vi "lockinOptimiser_old.vi"() -> ()   [LabVIEW 2014]
uses:
  <vilib>/Utility/file.llb/Read From Spreadsheet File (DBL).vi
  <userlib>/Nanonis Prog Interface V5/Nanonis Prog Interface.lvlib
  <vilib>/Analysis/NI_AALBase.lvlib
panel:
  in  "stop":bool
  in  "Start":bool
  in  "Clear Chart":bool
  in  "End Index":dbl=351.0
  in  "Start Index":dbl=250.0
  out "SNR":cluster{"all rows":dbl[], dbl[]}[](graph)
  out "Demod":cluster{"all rows":dbl[], dbl[]}[](graph)
  out "Std Dev Demod":cluster{"all rows":dbl[], dbl[]}[](graph)
  in  "Settling Time (ms)":i32=1000
  in  "Integration Time (ms)":i32=600
  out "all rows":dbl[][](array[numeric]) format="%0.3f"
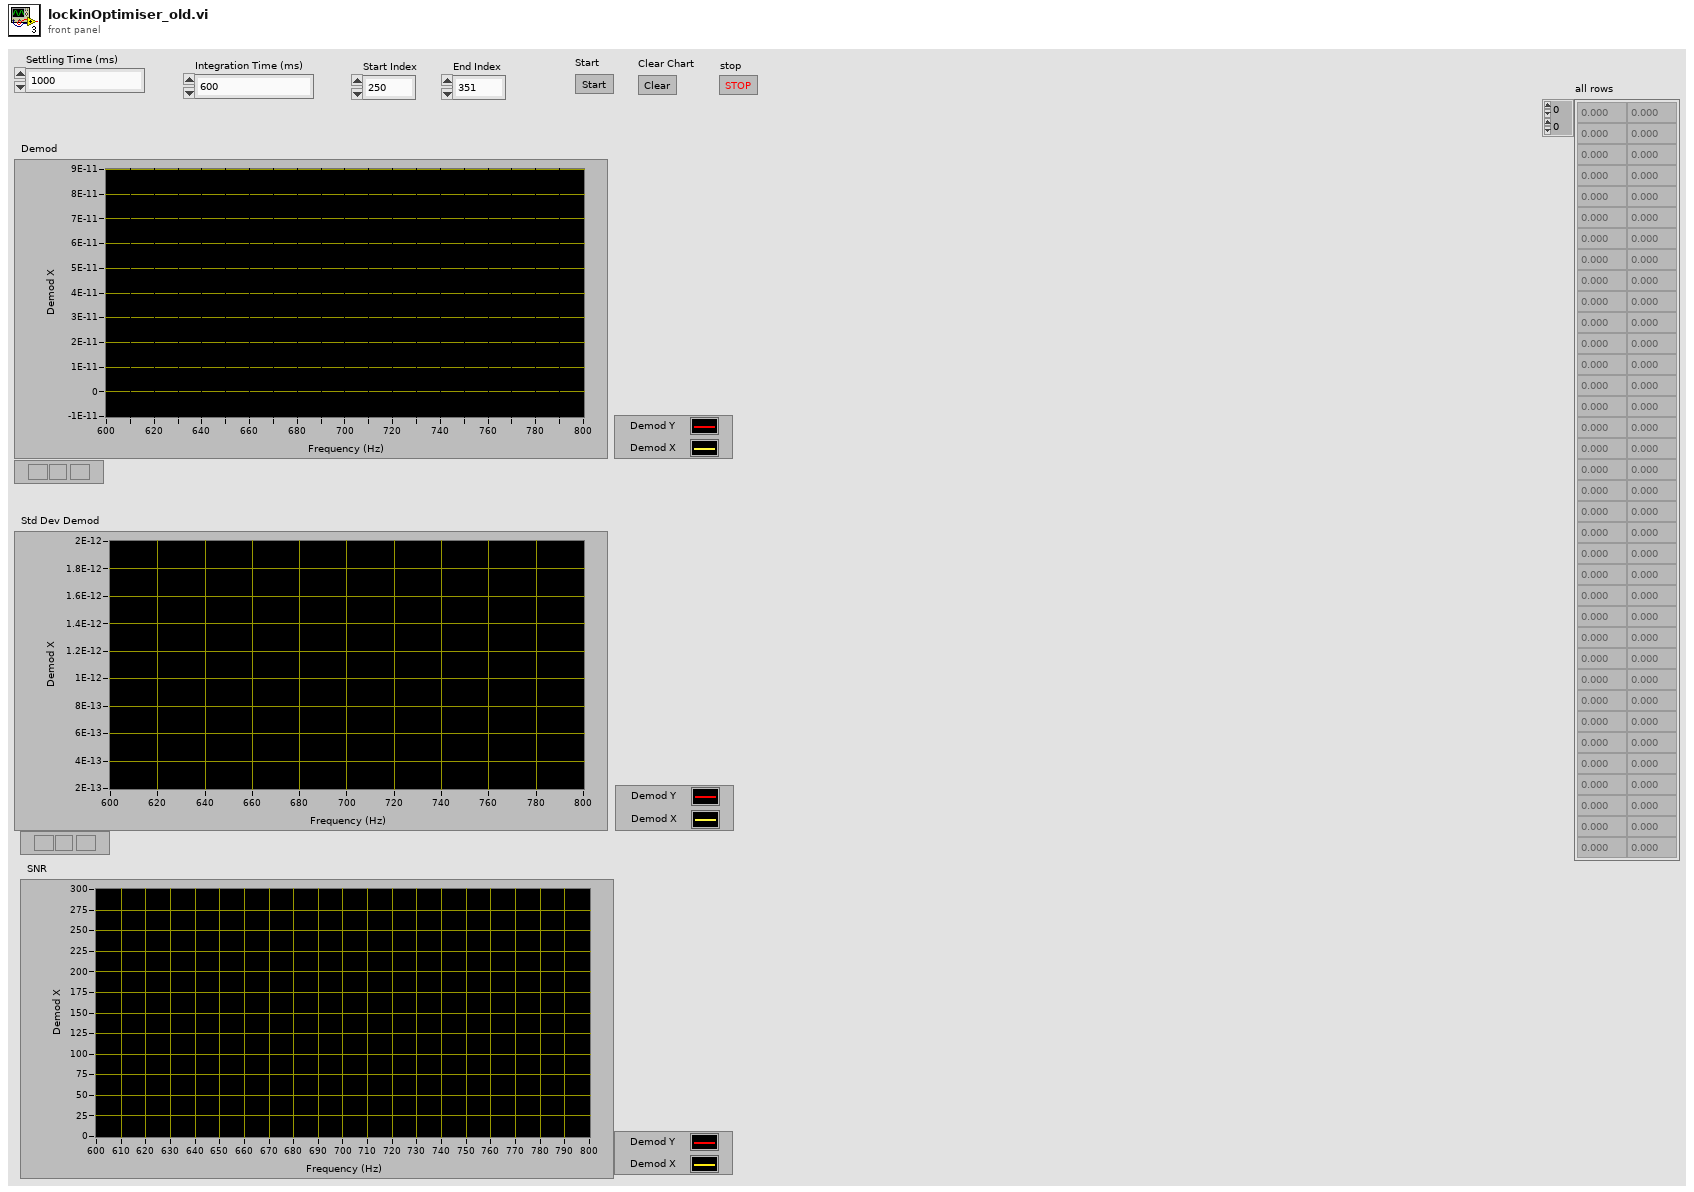
[diagram p1: front panel]
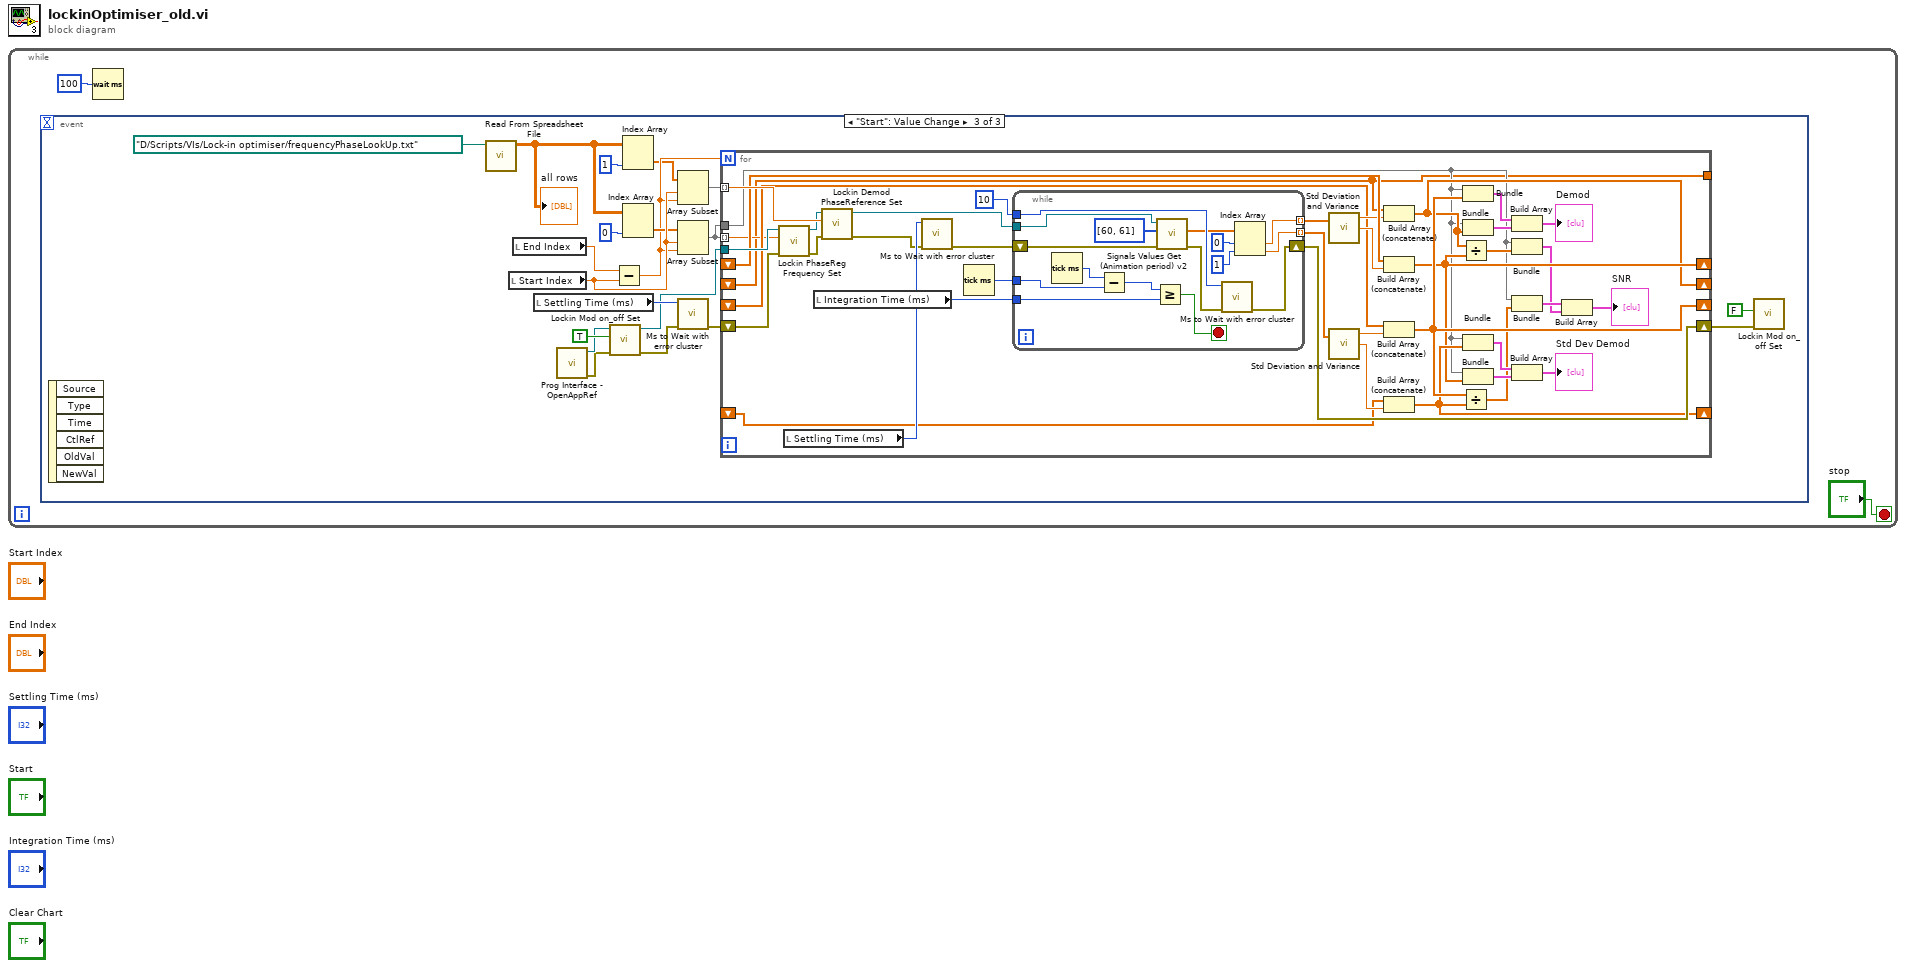
[diagram p0: block diagram]
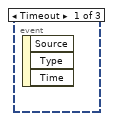
[diagram p2: hidden frame]
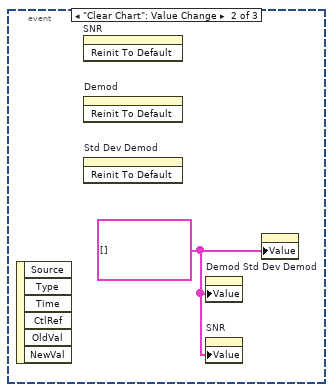
[diagram p3: hidden frame]
diagram:
  n1 = while {
    stop <- "stop" stop-if-true
    n2 = event shown="[2] \"Start\": Value Change" {
      selector: _ -> [_ _ _]
      dyn-events: _ -> [_ _ _]
      timeout: _ -> [_ _ _]
      event Timeout {
        n3 = event-data() -> ()  [unwired: 1 in, 3 out]
      }
      event "Clear Chart": Value Change {
        w3 = cluster{"all rows":dbl[], dbl[]}[] [] ("Demod")
        n4 = event-data() -> ()  [unwired: 1 in, 6 out]
        n5 = invoke on="SNR" class="XYGraph (strict)" method="Reinit To Default"() -> ()  [unwired: 3 in, 3 out]
        n6 = invoke on="Demod" class="XYGraph (strict)" method="Reinit To Default"() -> ()  [unwired: 3 in, 3 out]
        n7 = invoke on="Std Dev Demod" class="XYGraph (strict)" method="Reinit To Default"() -> ()  [unwired: 3 in, 3 out]
        n8 = property on="Demod" class="XYGraph (strict)"("Value"=w3) -> ()  [unwired: 2 in, 2 out]
        n9 = property on="SNR" class="XYGraph (strict)"("Value"=w3) -> ()  [unwired: 2 in, 2 out]
        n10 = property on="Std Dev Demod" class="XYGraph (strict)"("Value"=w3) -> ()  [unwired: 2 in, 2 out]
      }
      event "Start": Value Change {
        n11 = event-data() -> ()  [unwired: 1 in, 6 out]
        n12 = call-poly <vilib>:"Read From Spreadsheet File.vi"("file path (dialog if empty)"=path "D:/Scripts/VIs/Lock-in optimiser/frequencyPhaseLookUp.txt") -> ("all rows"=w7:dbl[][])  [unwired: 6 in, 4 out]
        "all rows" <- w7
        n13 = local read "Start Index"() -> (w22:dbl)
        n14 = local read "End Index"() -> (w23:dbl)
        n15 = local read "Settling Time (ms)"() -> (w21:i32)
        n16 = call <userlib>:"Prog Interface - OpenAppRef.vi"() -> ("Error out"=w8:errorcluster, "Application reference"=w9:refnum<vi>)  [unwired: 6 in]
        n17 = call <userlib>:"Lockin Mod on_off Set.vi"("Error in (no error)"=w8, "Lockin ON/OFF"=TRUE, "Application ref in"=w9) -> ("Error out"=w11:errorcluster, "Application ref out"=w10:refnum<vi>)  [unwired: 7 in]
        n18 = Subtract(x=w23, y=w22) -> (x-y=w17:dbl)
        n19 = Index Array(array=w7, index (col)=1 ("index")) -> (element=w16:dbl[])  [unwired: 1 in]
        n20 = Index Array(array=w7, index (col)=0 ("index")) -> (element=w18:dbl[])  [unwired: 1 in]
        n21 = Array Subset(array=w16, index=w22, length=w17) -> (w20:dbl[])
        n22 = Array Subset(array=w18, index=w22, length=w17) -> (w19:dbl[])
        n23 = call <userlib>:"Ms to Wait with error cluster.vi"("error in (no error)"=w11, "milliseconds to wait"=w21) -> ("error out"=w12:errorcluster)  [unwired: 4 in, 1 out]
        n24 = for {
          N: w17 -> [_]
          tunnel: w19 -> [w41] mode=indexing
          tunnel: w20 -> [w63] mode=indexing
          tunnel: w10 -> [w62]
          shift-right: [w51] -> w14
          shift-left: w12 -> [w60]
          shift-right: [w32] -> _
          shift-left: _ -> [w48]
          shift-right: [w31] -> _
          shift-left: _ -> [w24]
          shift-right: [w34] -> _
          shift-left: _ -> [w44]
          shift-right: [w33] -> _
          shift-left: _ -> [w42]
          tunnel: w19 -> [w28]
          tunnel: [w24] -> _
          n25 = call <userlib>:"Lockin PhaseReg Frequency Set.vi"("Error in (no error)"=w60, "Frequency (Hz)"=w41, "Application ref in"=w62) -> ("Error out"=w59:errorcluster, "Application ref out"=w61:refnum<vi>)  [unwired: 7 in]
          n26 = local read "Settling Time (ms)"() -> (w54:i32)
          n27 = local read "Integration Time (ms)"() -> (w55:i32)
          n28 = call <userlib>:"Lockin Demod PhaseReference Set.vi"("Error in (no error)"=w59, "Phase Reference"=w63, "Application ref in"=w61) -> ("Error out"=w53:errorcluster, "Application ref out"=w52:refnum<vi>)  [unwired: 7 in]
          n29 = call <userlib>:"Ms to Wait with error cluster.vi"("error in (no error)"=w53, "milliseconds to wait"=w54) -> ("error out"=w58:errorcluster)  [unwired: 4 in, 1 out]
          n30 = Tick Count (ms)() -> (millisecond timer value=w57:u32)
          n31 = while {
            tunnel: w57 -> [w79]
            tunnel: 10 ("Integration Time (ms)") -> [w75]
            tunnel: w55 -> [w74]
            tunnel: w52 -> [w72]
            tunnel: [w65] -> w50 mode=indexing
            tunnel: [w64] -> w49 mode=indexing
            shift-right: [w73] -> w51
            shift-left: w58 -> [w71]
            stop <- w76 stop-if-true
            n32 = Tick Count (ms)() -> (millisecond timer value=w78:u32)
            n33 = Subtract(x=w78, y=w79) -> (x-y=w77:u32)
            n34 = Greater Or Equal?(x=w77, y=w74) -> (x >= y?=w76:bool)
            n35 = call <userlib>:"Signals Values Get (Animation period) v2.vi"("error in (no error)"=w71, "Signals indexes (0-79)"=i8[] [60, 61], "Application ref in"=w72) -> ("error out"=w70:errorcluster, "Signals Values"=w68:sgl[])  [unwired: 5 in, 1 out]
            n36 = call <userlib>:"Ms to Wait with error cluster.vi"("error in (no error)"=w70, "milliseconds to wait"=w75) -> ("error out"=w73:errorcluster)  [unwired: 4 in, 1 out]
            n37 = Index Array(array=w68, index #1=0 ("index"), index #2=1 ("index")) -> (element #1=w65:sgl, element #2=w64:sgl)
          }
          n38 = call <vilib>:"Std Deviation and Variance.vi"("X"=w50) -> ("mean"=w46:dbl, "standard deviation"=w47:dbl)  [unwired: 1 in, 1 out]
          n39 = call <vilib>:"Std Deviation and Variance.vi"("X"=w49) -> ("mean"=w45:dbl, "standard deviation"=w43:dbl)  [unwired: 1 in, 1 out]
          n40 = Build Array (concatenate)(w24, w46) -> (w31:dbl[])
          n41 = Build Array (concatenate)(w48, w47) -> (w32:dbl[])
          n42 = Build Array (concatenate)(w44, w45) -> (w34:dbl[])
          n43 = Build Array (concatenate)(w42, w43) -> (w33:dbl[])
          n44 = Divide(x=w31, y=w32) -> (x/y=w29:dbl[])
          n45 = Divide(x=w34, y=w33) -> (x/y=w30:dbl[])
          n46 = Bundle(w28, w34) -> (w39:cluster{dbl[], dbl[]})  [unwired: 1 in]
          n47 = Bundle(w28, w31) -> (w38:cluster{dbl[], dbl[]})  [unwired: 1 in]
          n48 = Bundle(w28, w33) -> (w36:cluster{dbl[], dbl[]})  [unwired: 1 in]
          n49 = Bundle(w28, w32) -> (w37:cluster{dbl[], dbl[]})  [unwired: 1 in]
          n50 = Build Array(w39, w38) -> (→"Demod":cluster{dbl[], dbl[]}[])
          n51 = Bundle(w28, w29) -> (w26:cluster{dbl[], dbl[]})  [unwired: 1 in]
          n52 = Bundle(w28, w30) -> (w27:cluster{dbl[], dbl[]})  [unwired: 1 in]
          n53 = Build Array(w36, w37) -> (→"Std Dev Demod":cluster{dbl[], dbl[]}[])
          n54 = Build Array(w27, w26) -> (→"SNR":cluster{dbl[], dbl[]}[])
        }
        n55 = call <userlib>:"Lockin Mod on_off Set.vi"("Error in (no error)"=w14, "Lockin ON/OFF"=FALSE) -> ()  [unwired: 8 in, 2 out]
      }
    }
    n56 = Wait (ms)(milliseconds to wait=u32 100) -> ()  [unwired: 1 out]
  }
